vi "Z6CSMain.contents.vi"   [LabVIEW 2014, in "Z6CSMain.lvlib"]
doc: "This class is forseen to select Z6 devices to work with. Therefore it reads the data base. It also opens a connection to other Z6 or PCS nodes.\n\nThis class is part of the Z6 resp. PHELIX user layer."
uses:
  Z6CSMain.lvlib
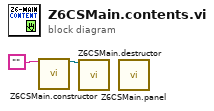
[diagram p0: block diagram]
diagram:
  n1 = call "Z6CSMain.constructor.vi"("name"="") -> ("i ref out"=w1:refnum<vi>)  [unwired: 16 in, 2 out]
  n2 = call "Z6CSMain.destructor.vi"("i ref in"=w1) -> ()  [unwired: 18 in, 1 out]
  n3 = call "Z6CSMain.panel.vi"() -> ()  [unwired: 19 in, 1 out]
